vi "Color Get CRI Hires.vi"(0 "a_data":dbl[](array[numeric]), 1 "a_NumPoints":u16, 2 "a_Observer":u8, 3 "a_samplenumber":u8, 4 "a_xarray":dbl[](array[numeric]), 5 "a_yarray":dbl[](array[numeric]), 6 "a_zarray":dbl[](array[numeric]), 7 "a_Rvalue":dbl, 8 "a_CRItable":dbl[](array[numeric]), 9 "error in (no error)":errorcluster) -> (11 "error out":errorcluster, 13 "a_Rvalue out":dbl, 14 "a_data out":dbl[](array[numeric]), 15 "function return":i16, 16 "a_xarray out":dbl[](array[numeric]), 17 "a_yarray out":dbl[](array[numeric]), 18 "a_zarray out":dbl[](array[numeric]), 19 "a_CRItable out":dbl[](array[numeric]))   [LabVIEW 2013, in "AVSirrad.lvlib"]
doc: "DLL_API short int __stdcall Color_GetColorRenderingIndex\n(\n DataType *a_data,\n unsigned char a_CIEResolution,\n unsigned char a_Observer,\n double *R_Values,\n double *CRI\n);"
uses:
  AVSirrad.lvlib
  AVSIRRAD/Examples/Labview/build/AVSirrad.dll
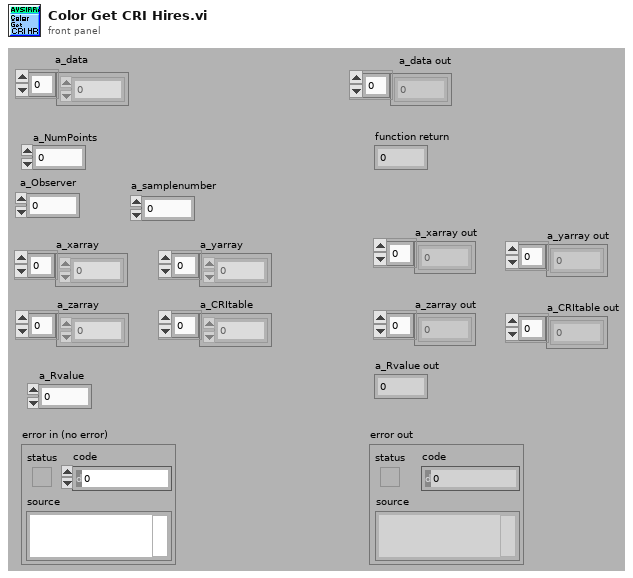
[diagram p1: front panel]
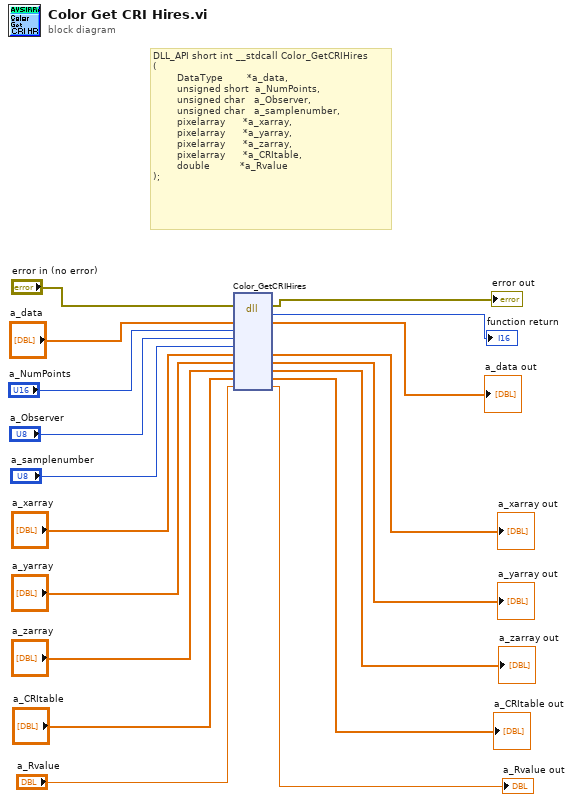
[diagram p0: block diagram]
diagram:
  # "DLL_API short int __stdcall Color_GetCRIHires\n(\n        DataType        *a_data,\n        unsigned short  a_NumPoints,\n        unsigned char   a_Observer,\n        unsigned char   a_samplenumber,\n        pixelarray      *a_xarray,\n        pixelarray      *a_yarray,\n        pixelarray      *a_zarray,\n        pixelarray      *a_CRItable,\n        double          *a_Rvalue\n);"
  n1 = dll-call lib="C:/AVSIRRAD/Examples/Labview/build/AVSirrad.*" fn="Color_GetCRIHires"(error in="error in (no error)", "a_data"="a_data", "a_NumPoints"="a_NumPoints", "a_Observer"="a_Observer", "a_samplenumber"="a_samplenumber", "a_xarray"="a_xarray", "a_yarray"="a_yarray", "a_zarray"="a_zarray", "a_CRItable"="a_CRItable", "a_Rvalue"="a_Rvalue") -> (error out=→"error out":errorcluster, "return type"=→"function return":i16, "a_data"=→"a_data out":dbl[], "a_xarray"=→"a_xarray out":dbl[], "a_yarray"=→"a_yarray out":dbl[], "a_zarray"=→"a_zarray out":dbl[], "a_CRItable"=→"a_CRItable out":dbl[], "a_Rvalue"=→"a_Rvalue out":dbl)  [unwired: 5 in, 1 out]
